vi "NR Fetch ACP.vi"(0 "RFmx Handle In":refnum<k21>, 1 "Selector String":string, 11 "error in (no error)":errorcluster) -> (4 "RFmx Handle Out":refnum<k21>, 6 "ACP Results":T1, 15 "error out":errorcluster)   [LabVIEW 2019, in "RFmxNR.lvlib"]
doc: "Fetches common results from the ACP measurement."
uses:
  RFmxNR.lvlib
  Typedefs/NR ACP Results.ctl
  Typedefs/NR ACP Offset Results.ctl
  Typedefs/NR ACP Component Carrier Results.ctl
  <vilib>/RFmx/NR/mx/RFmxNR.llb/RFmxNR ACP Fetch Offset Measurement (Array).vi
  <vilib>/RFmx/NR/mx/RFmxNR.llb/RFmxNR ACP Fetch Component Carrier Measurement (Array).vi
  <resource>/objmgr/RFmxNR.rc
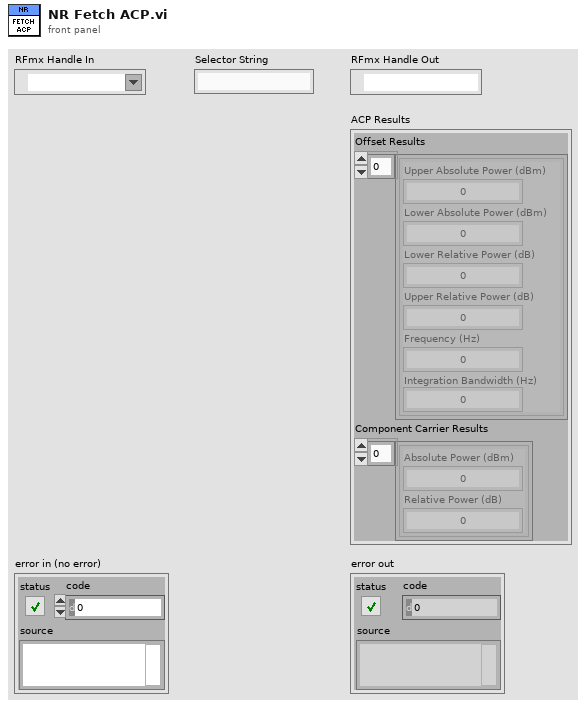
[diagram p1: front panel]
types:
  T1 = typedef "RFmxNR.lvlib/NR ACP Results.ctl" = cluster{"Offset Results":T2[], "Component Carrier Results":T3[]}
  T2 = typedef "RFmxNR.lvlib/NR ACP Offset Results.ctl" = cluster{"Upper Absolute Power (dBm)":dbl, "Lower Absolute Power (dBm)":dbl, "Lower Relative Power (dB)":dbl, "Upper Relative Power (dB)":dbl, "Frequency (Hz)":dbl, "Integration Bandwidth (Hz)":dbl}
  T3 = typedef "RFmxNR.lvlib/NR ACP Component Carrier Results.ctl" = cluster{"Absolute Power (dBm)":dbl, "Relative Power (dB)":dbl}
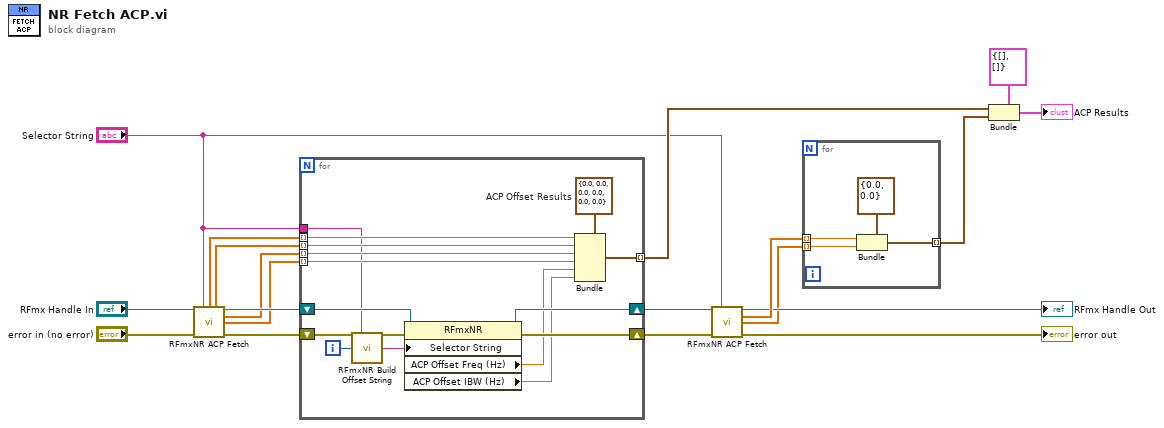
[diagram p0: block diagram]
diagram:
  n1 = call-poly <vilib>:"RFmxNR ACP Fetch.vi"("Instrument Handle In"="RFmx Handle In", "Selector String"="Selector String", "error in (no error)"="error in (no error)") -> ("Upper Absolute Power (dBm)"=w5:dbl[], "Lower Absolute Power (dBm)"=w15:dbl[], "Instrument Handle Out"=w17:refnum<k21>, "Lower Relative Power (dB)"=w14:dbl[], "Upper Relative Power (dB)"=w13:dbl[], "error out"=w16:errorcluster)  [unwired: 7 in]
  n2 = for {
    shift-right: [w32] -> w12
    shift-left: w17 -> [w28]
    shift-right: [w33] -> w11
    shift-left: w16 -> [w27]
    tunnel: [w30] -> w18 mode=indexing
    tunnel: w5 -> [w26] mode=indexing
    tunnel: w15 -> [w25] mode=indexing
    tunnel: w14 -> [w24] mode=indexing
    tunnel: w13 -> [w23] mode=indexing
    tunnel: "Selector String" -> [w22]
    i -> [w34]
    w31 = T2 {"Upper Absolute Power (dBm)"=0.0, "Lower Absolute Power (dBm)"=0.0, "Lower Relative Power (dB)"=0.0, "Upper Relative Power (dB)"=0.0, "Frequency (Hz)"=0.0, "Integration Bandwidth (Hz)"=0.0}  # ACP Offset Results
    n3 = call <vilib>:"RFmxNR Build Offset String.vi"("Selector String"=w22, "Offset Number"=w34) -> ("Selector String Out"=w29:string)  [unwired: 13 in]
    n4 = property class="RFmxNR"(reference=w28, error in=w27, "Selector String"=w29) -> (reference out=w32:refnum<k21>, error out=w33:errorcluster, "ACP Offset Freq (Hz)"=w20:dbl, "ACP Offset IBW (Hz)"=w21:dbl)
    n5 = Bundle(cluster=w31, "Upper Absolute Power (dBm)"=w26, "Lower Absolute Power (dBm)"=w25, "Lower Relative Power (dB)"=w24, "Upper Relative Power (dB)"=w23, "Frequency (Hz)"=w20, "Integration Bandwidth (Hz)"=w21) -> (w30:T2)
  }
  n6 = call-poly <vilib>:"RFmxNR ACP Fetch.vi"("Instrument Handle In"=w12, "Selector String"="Selector String", "error in (no error)"=w11) -> ("Instrument Handle Out"=→"RFmx Handle Out":refnum<k21>, "Absolute Power (dBm)"=w10:dbl[], "Relative Power (dB)"=w4:dbl[], "error out"=→"error out":errorcluster)  [unwired: 9 in]
  n7 = for {
    tunnel: [w38] -> w19 mode=indexing
    tunnel: w10 -> [w37] mode=indexing
    tunnel: w4 -> [w36] mode=indexing
    n8 = Bundle(cluster=T3 {"Absolute Power (dBm)"=0.0, "Relative Power (dB)"=0.0} ("NR ACP Component Carrier Results"), "Absolute Power (dBm)"=w37, "Relative Power (dB)"=w36) -> (w38:T3)
  }
  n9 = Bundle(cluster=T1 {"Offset Results"=[], "Component Carrier Results"=[]} ("NR ACP Results"), "Offset Results"=w18, "Component Carrier Results"=w19) -> (→"ACP Results":T1)
